vi "Set HTTP Server Info.vi"(8 "error in (no error)":errorcluster, 10 "HTTP Server Info":T1, 11 "Node Config in":refnum<class "Node Config.lvclass">) -> (0 "error out":errorcluster, 3 "Node Config out":refnum<class "Node Config.lvclass">)   [LabVIEW 2020, in "Vecto.lvlib" / "Node Config.lvclass"]
uses:
  Node Config.lvclass
  Node Config.lvclass/Node Config.ctl
  HTTP Server Info.ctl
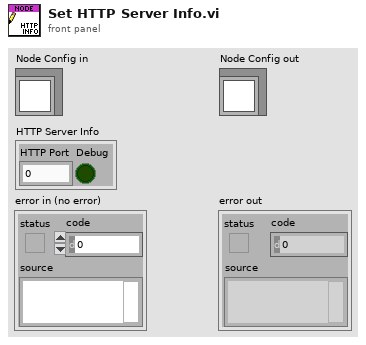
[diagram p1: front panel]
types:
  T1 = typedef "Vecto.lvlib/Node Config.lvclass/HTTP Server Info.ctl" = cluster{"HTTP Port":u16, "Debug":bool}
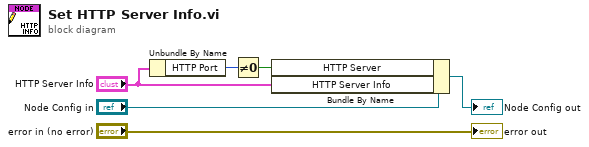
[diagram p0: block diagram]
diagram:
  n1 = Unbundle By Name("HTTP Server Info") -> ("HTTP Port"=w2:u16)
  n2 = Not Equal To 0?(x=w2) -> (x != 0?=w1:bool)
  n3 = Bundle By Name(cluster="Node Config in", "HTTP Server"=w1, "HTTP Server Info"="HTTP Server Info") -> (→"Node Config out":refnum<class "Node Config.lvclass">)
  "error out" <- "error in (no error)"
